vi "DatabaseAPI-UpdateNull.vi"(0 "Database-API in":refnum<class "Database-API.lvclass">, 1 "data":variant, 2 "Where Statement":string, 3 "Columns":string, 5 "Update All":bool, 7 "Table":string, 9 "Column Number":i32, 11 "error in (no error)":errorcluster, 14 "IS NULL":bool) -> (4 "Database-API out":refnum<class "Database-API.lvclass">, 15 "error out":errorcluster)   [LabVIEW 2014, in "Database-API.lvclass"]
uses:
  Database-API.lvclass
  <vilib>/addons/database/NI_Database_API.lvlib
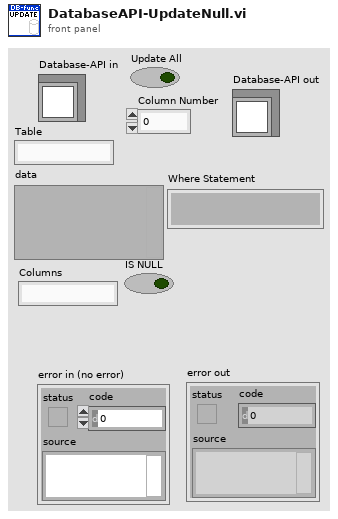
[diagram p1: front panel]
types:
  T1 = typedef "NI_Database_API.lvlib/Conn ObjectReference.ctl" = refnum<k1>
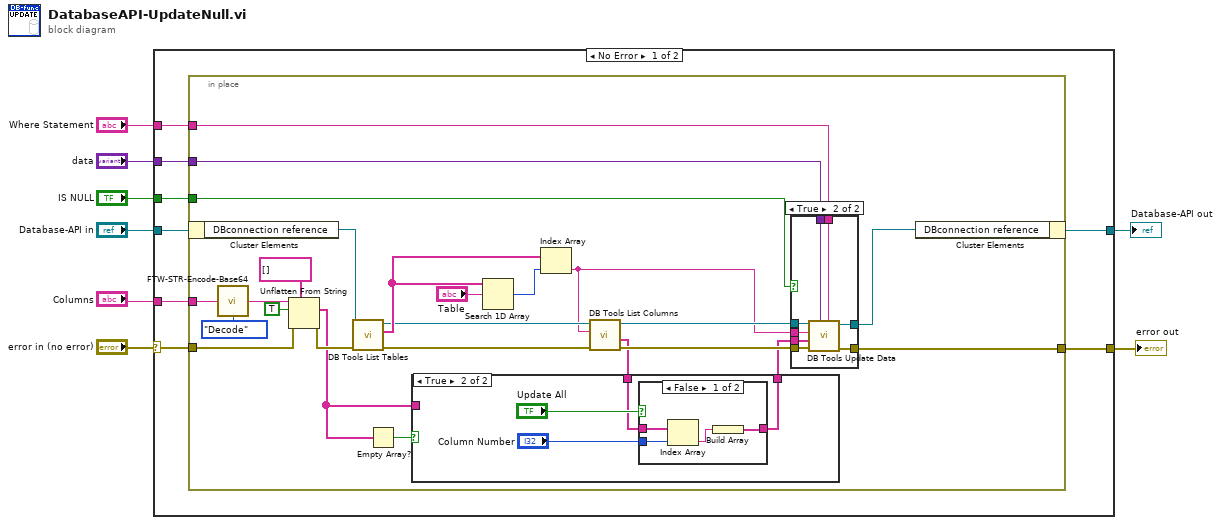
[diagram p0: block diagram]
diagram:
  n1 = case shown="No Error" "error in (no error)" {
    selector: "error in (no error)" -> [w14 w61]
    tunnel: [w13 w61] -> w7
    tunnel: [w15 w60] -> w5
    tunnel: "Database-API in" -> [w16 w60]
    tunnel: "Columns" -> [w12 _]
    tunnel: "data" -> [w11 _]
    tunnel: "Where Statement" -> [w10 _]
    tunnel: "IS NULL" -> [w9 _]
    frame No Error {
      n2 = in-place {
        in-place-border: w14 -> [w20]
        in-place-border: [w29] -> w13
        in-place-border: w12 -> [w21]
        in-place-border: w11 -> [w27]
        in-place-border: w10 -> [w26]
        in-place-border: w9 -> [w17]
        n3 = in-place-cluster #1(w16) -> ("DBconnection reference"=w41:T1)
        n4 = call "FTW-STR-Encode-Base64.vi"("Input"=w21, "Direction"=enum16{"Encode", "Decode"}."Decode") -> ("Output"=w23:string)
        n5 = Unflatten From String(type=string[] [] ("Columns"), binary string=w23, data includes array or string size? (T)=TRUE, error in (no error)=w20) -> (value=w18:string[], error out=w19:errorcluster)  [unwired: 1 in, 1 out]
        n6 = call <vilib>:"DB Tools List Tables.vi"("error in (no error)"=w19, "connection reference"=w41) -> ("error out"=w37:errorcluster, "tables"=w40:string[], "connection reference out"=w36:T1)  [unwired: 3 in]
        n7 = Empty Array?(array=w18) -> (empty?=w28:bool)
        n8 = Search 1D Array(1D array=w40, element="Table") -> (index of element=w38:i32)  [unwired: 1 in]
        n9 = Index Array(array=w40, index=w38) -> (element=w31:string)
        n10 = call <vilib>:"DB Tools List Columns.vi"("error in (no error)"=w37, "table"=w31, "connection reference"=w36) -> ("error out"=w35:errorcluster, "columns"=w33:string[], "connection reference out"=w34:T1)  [unwired: 1 in, 1 out]
        n11 = case shown="True" w28 {
          tunnel: w33 -> [_ w53]
          tunnel: [w50 w52] -> w32
          tunnel: w18 -> [w50 _]
          frame False {
          }
          frame True {
            n12 = case shown="False" "Update All" {
              tunnel: w53 -> [w58 w59]
              tunnel: [w55 w59] -> w52
              tunnel: "Column Number" -> [w57 _]
              frame False {
                n13 = Index Array(array=w58, index=w57) -> (element=w56:string)
                n14 = Build Array(w56) -> (w55:string[])
              }
              frame True {
              }
            }
          }
        }
        n15 = case shown="True" w17 {
          tunnel: w35 -> [_ w49]
          tunnel: w34 -> [_ w48]
          tunnel: w32 -> [_ w47]
          tunnel: w31 -> [_ w46]
          tunnel: [_ w45] -> w30
          tunnel: [_ w44] -> w29
          tunnel: w27 -> [_ w43]
          tunnel: w26 -> [_ w42]
          frame False {
          }
          frame True {
            n16 = call <vilib>:"DB Tools Update Data.vi"("condition"=w42, "data"=w43, "error in (no error)"=w49, "columns"=w47, "table"=w46, "connection reference"=w48) -> ("error out"=w44:errorcluster, "connection reference out"=w45:T1)  [unwired: 4 in]
          }
        }
        n17 = in-place-cluster #1("DBconnection reference"=w30) -> (w15:refnum<class "Database-API.lvclass">)
      }
    }
    frame Error {
    }
  }
  "error out" <- w7
  "Database-API out" <- w5
